vi "Lab Panel V5.12.vi"() -> ()   [LabVIEW 2013] (continued)
                    }
                    n1129 = Increment(x=w2161) -> (x+1=w2162:dbl)
                    n1130 = Greater Or Equal?(x=w2169, y=w2162) -> (x >= y?=w2171:bool)
                    n1131 = case shown="True" w2171 {
                      tunnel: w2166 -> [w2181 _]
                      tunnel: w2165 -> [w2180 _]
                      tunnel: w2164 -> [w2179 _]
                      tunnel: w2163 -> [w2178 _]
                      frame True {
                        n1132 = stacked-sequence {
                          tunnel: w2181 -> [w2185 _]
                          tunnel: w2180 -> [w2183 w2189]
                          tunnel: w2179 -> [_ w2192]
                          tunnel: w2178 -> [w2182 _]
                          frame #0 {
                            n1133 = Build Array(w2183) -> (w2186:string[])
                            n1134 = Build Array(w2185) -> (w2184:dbl[])
                            n1135 = TDMS Write(0:w2182, 5:"TEST PASS", 7:w2186, 9:w2184) -> (15:w2188:errorcluster)  [unwired: 2 in, 3 out]
                            n1136 = local write "data file error"(w2188) -> ()
                          }
                          frame #1 {
                            n1137 = Bundle(cluster=w2192, "STATUS"=w2189) -> (w2190:T4)  [unwired: 2 in]
                            n1138 = local write "RESULT LAB02-1"(TRUE) -> ()
                            n1139 = local write "DISP LAB02-1"(w2190) -> ()
                          }
                        }
                      }
                      frame False {
                      }
                    }
                  }
                }
              }
              frame #3 {
                # "LAB02-2"
                n1140 = Less?(x=w2193, y=2) -> (x < y?=w2196:bool)
                n1141 = local read "DISP LAB02-2"() -> (w2198:T4)
                n1142 = Unbundle(w2198) -> ("STATUS"=w2199:string)  [unwired: 2 out]
                n1143 = Equal?(x=w2199, y="RUN") -> (x = y?=w2195:bool)
                n1144 = And(x=w2195, y=w2196) -> (x .and. y?=w2194:bool)
                n1145 = case shown="True" w2194 {
                  tunnel: w2198 -> [_ w2204]
                  tunnel: w2193 -> [_ w2208]
                  frame False {
                  }
                  frame True {
                    n1146 = local read "SET LAB02-2"() -> (w2210:T5)
                    n1147 = local read "TDMS LAB02-2"() -> (w2203:refnum<k34>)
                    n1148 = Unbundle(w2204) -> ("CYCLE"=w2209:dbl)  [unwired: 2 out]
                    n1149 = Unbundle(w2210) -> ("CYCLES"=w2201:dbl, "T-RISE mins"=w2207:dbl)  [unwired: 3 out]
                    n1150 = case shown="\"T-RISE TEST\"" w2208 {
                      tunnel: w2207 -> [_ _ w2217]
                      tunnel: [w2212 w2214 w2217] -> w2206
                      tunnel: w2201 -> [w2212 w2214 _]
                      tunnel: ["CHART PASS" "CYCLE PASS" "T-RISE PASS"] -> w2205
                      frame "CHART TEST", Default {
                      }
                      frame "CYCLE TEST" {
                      }
                      frame "T-RISE TEST" {
                      }
                    }
                    n1151 = Increment(x=w2201) -> (x+1=w2202:dbl)
                    n1152 = Greater Or Equal?(x=w2209, y=w2202) -> (x >= y?=w2211:bool)
                    n1153 = case shown="True" w2211 {
                      tunnel: w2206 -> [w2221 _]
                      tunnel: w2205 -> [w2220 _]
                      tunnel: w2204 -> [w2219 _]
                      tunnel: w2203 -> [w2218 _]
                      frame True {
                        n1154 = stacked-sequence {
                          tunnel: w2221 -> [w2225 _]
                          tunnel: w2220 -> [w2223 w2229]
                          tunnel: w2219 -> [_ w2232]
                          tunnel: w2218 -> [w2222 _]
                          frame #0 {
                            n1155 = Build Array(w2223) -> (w2226:string[])
                            n1156 = Build Array(w2225) -> (w2224:dbl[])
                            n1157 = TDMS Write(0:w2222, 5:"TEST PASS", 7:w2226, 9:w2224) -> (15:w2228:errorcluster)  [unwired: 2 in, 3 out]
                            n1158 = local write "data file error"(w2228) -> ()
                          }
                          frame #1 {
                            n1159 = Bundle(cluster=w2232, "STATUS"=w2229) -> (w2230:T4)  [unwired: 2 in]
                            n1160 = local write "RESULT LAB02-2"(TRUE) -> ()
                            n1161 = local write "DISP LAB02-2"(w2230) -> ()
                          }
                        }
                      }
                      frame False {
                      }
                    }
                  }
                }
              }
              frame #4 {
                # "LAB03-1"
                n1162 = Less?(x=w2233, y=2) -> (x < y?=w2236:bool)
                n1163 = local read "DISP LAB03-1"() -> (w2238:T4)
                n1164 = Unbundle(w2238) -> ("STATUS"=w2239:string)  [unwired: 2 out]
                n1165 = Equal?(x=w2239, y="RUN") -> (x = y?=w2235:bool)
                n1166 = And(x=w2235, y=w2236) -> (x .and. y?=w2234:bool)
                n1167 = case shown="True" w2234 {
                  tunnel: w2238 -> [_ w2244]
                  tunnel: w2233 -> [_ w2248]
                  frame False {
                  }
                  frame True {
                    n1168 = local read "SET LAB03-1"() -> (w2250:T5)
                    n1169 = local read "TDMS LAB03-1"() -> (w2243:refnum<k34>)
                    n1170 = Unbundle(w2244) -> ("CYCLE"=w2249:dbl)  [unwired: 2 out]
                    n1171 = Unbundle(w2250) -> ("CYCLES"=w2241:dbl, "T-RISE mins"=w2247:dbl)  [unwired: 3 out]
                    n1172 = case shown="\"T-RISE TEST\"" w2248 {
                      tunnel: w2247 -> [_ _ w2257]
                      tunnel: [w2252 w2254 w2257] -> w2246
                      tunnel: w2241 -> [w2252 w2254 _]
                      tunnel: ["CHART PASS" "CYCLE PASS" "T-RISE PASS"] -> w2245
                      frame "CHART TEST", Default {
                      }
                      frame "CYCLE TEST" {
                      }
                      frame "T-RISE TEST" {
                      }
                    }
                    n1173 = Increment(x=w2241) -> (x+1=w2242:dbl)
                    n1174 = Greater Or Equal?(x=w2249, y=w2242) -> (x >= y?=w2251:bool)
                    n1175 = case shown="True" w2251 {
                      tunnel: w2246 -> [w2261 _]
                      tunnel: w2245 -> [w2260 _]
                      tunnel: w2244 -> [w2259 _]
                      tunnel: w2243 -> [w2258 _]
                      frame True {
                        n1176 = stacked-sequence {
                          tunnel: w2261 -> [w2265 _]
                          tunnel: w2260 -> [w2263 w2269]
                          tunnel: w2259 -> [_ w2272]
                          tunnel: w2258 -> [w2262 _]
                          frame #0 {
                            n1177 = Build Array(w2263) -> (w2266:string[])
                            n1178 = Build Array(w2265) -> (w2264:dbl[])
                            n1179 = TDMS Write(0:w2262, 5:"TEST PASS", 7:w2266, 9:w2264) -> (15:w2268:errorcluster)  [unwired: 2 in, 3 out]
                            n1180 = local write "data file error"(w2268) -> ()
                          }
                          frame #1 {
                            n1181 = Bundle(cluster=w2272, "STATUS"=w2269) -> (w2270:T4)  [unwired: 2 in]
                            n1182 = local write "RESULT LAB03-1"(TRUE) -> ()
                            n1183 = local write "DISP LAB03-1"(w2270) -> ()
                          }
                        }
                      }
                      frame False {
                      }
                    }
                  }
                }
              }
              frame #5 {
                # "LAB03-2"
                n1184 = Less?(x=w2273, y=2) -> (x < y?=w2276:bool)
                n1185 = local read "DISP LAB03-2"() -> (w2278:T4)
                n1186 = Unbundle(w2278) -> ("STATUS"=w2279:string)  [unwired: 2 out]
                n1187 = Equal?(x=w2279, y="RUN") -> (x = y?=w2275:bool)
                n1188 = And(x=w2275, y=w2276) -> (x .and. y?=w2274:bool)
                n1189 = case shown="True" w2274 {
                  tunnel: w2278 -> [_ w2284]
                  tunnel: w2273 -> [_ w2288]
                  frame False {
                  }
                  frame True {
                    n1190 = local read "SET LAB03-2"() -> (w2290:T5)
                    n1191 = local read "TDMS LAB03-2"() -> (w2283:refnum<k34>)
                    n1192 = Unbundle(w2284) -> ("CYCLE"=w2289:dbl)  [unwired: 2 out]
                    n1193 = Unbundle(w2290) -> ("CYCLES"=w2281:dbl, "T-RISE mins"=w2287:dbl)  [unwired: 3 out]
                    n1194 = case shown="\"T-RISE TEST\"" w2288 {
                      tunnel: w2287 -> [_ _ w2297]
                      tunnel: [w2292 w2294 w2297] -> w2286
                      tunnel: w2281 -> [w2292 w2294 _]
                      tunnel: ["CHART PASS" "CYCLE PASS" "T-RISE PASS"] -> w2285
                      frame "CHART TEST", Default {
                      }
                      frame "CYCLE TEST" {
                      }
                      frame "T-RISE TEST" {
                      }
                    }
                    n1195 = Increment(x=w2281) -> (x+1=w2282:dbl)
                    n1196 = Greater Or Equal?(x=w2289, y=w2282) -> (x >= y?=w2291:bool)
                    n1197 = case shown="True" w2291 {
                      tunnel: w2286 -> [w2301 _]
                      tunnel: w2285 -> [w2300 _]
                      tunnel: w2284 -> [w2299 _]
                      tunnel: w2283 -> [w2298 _]
                      frame True {
                        n1198 = stacked-sequence {
                          tunnel: w2301 -> [w2305 _]
                          tunnel: w2300 -> [w2303 w2309]
                          tunnel: w2299 -> [_ w2312]
                          tunnel: w2298 -> [w2302 _]
                          frame #0 {
                            n1199 = Build Array(w2303) -> (w2306:string[])
                            n1200 = Build Array(w2305) -> (w2304:dbl[])
                            n1201 = TDMS Write(0:w2302, 5:"TEST PASS", 7:w2306, 9:w2304) -> (15:w2308:errorcluster)  [unwired: 2 in, 3 out]
                            n1202 = local write "data file error"(w2308) -> ()
                          }
                          frame #1 {
                            n1203 = Bundle(cluster=w2312, "STATUS"=w2309) -> (w2310:T4)  [unwired: 2 in]
                            n1204 = local write "RESULT LAB03-2"(TRUE) -> ()
                            n1205 = local write "DISP LAB03-2"(w2310) -> ()
                          }
                        }
                      }
                      frame False {
                      }
                    }
                  }
                }
              }
              frame #6 {
                # "LAB04-1"
                n1206 = Less?(x=w2313, y=2) -> (x < y?=w2316:bool)
                n1207 = local read "DISP LAB04-1"() -> (w2318:T4)
                n1208 = Unbundle(w2318) -> ("STATUS"=w2319:string)  [unwired: 2 out]
                n1209 = Equal?(x=w2319, y="RUN") -> (x = y?=w2315:bool)
                n1210 = And(x=w2315, y=w2316) -> (x .and. y?=w2314:bool)
                n1211 = case shown="True" w2314 {
                  tunnel: w2318 -> [_ w2324]
                  tunnel: w2313 -> [_ w2328]
                  frame False {
                  }
                  frame True {
                    n1212 = local read "SET LAB04-1"() -> (w2330:T5)
                    n1213 = local read "TDMS LAB04-1"() -> (w2323:refnum<k34>)
                    n1214 = Unbundle(w2324) -> ("CYCLE"=w2329:dbl)  [unwired: 2 out]
                    n1215 = Unbundle(w2330) -> ("CYCLES"=w2321:dbl, "T-RISE mins"=w2327:dbl)  [unwired: 3 out]
                    n1216 = case shown="\"T-RISE TEST\"" w2328 {
                      tunnel: w2327 -> [_ _ w2337]
                      tunnel: [w2332 w2334 w2337] -> w2326
                      tunnel: w2321 -> [w2332 w2334 _]
                      tunnel: ["CHART PASS" "CYCLE PASS" "T-RISE PASS"] -> w2325
                      frame "CHART TEST", Default {
                      }
                      frame "CYCLE TEST" {
                      }
                      frame "T-RISE TEST" {
                      }
                    }
                    n1217 = Increment(x=w2321) -> (x+1=w2322:dbl)
                    n1218 = Greater Or Equal?(x=w2329, y=w2322) -> (x >= y?=w2331:bool)
                    n1219 = case shown="True" w2331 {
                      tunnel: w2326 -> [w2341 _]
                      tunnel: w2325 -> [w2340 _]
                      tunnel: w2324 -> [w2339 _]
                      tunnel: w2323 -> [w2338 _]
                      frame True {
                        n1220 = stacked-sequence {
                          tunnel: w2341 -> [w2345 _]
                          tunnel: w2340 -> [w2343 w2349]
                          tunnel: w2339 -> [_ w2352]
                          tunnel: w2338 -> [w2342 _]
                          frame #0 {
                            n1221 = Build Array(w2343) -> (w2346:string[])
                            n1222 = Build Array(w2345) -> (w2344:dbl[])
                            n1223 = TDMS Write(0:w2342, 5:"TEST PASS", 7:w2346, 9:w2344) -> (15:w2348:errorcluster)  [unwired: 2 in, 3 out]
                            n1224 = local write "data file error"(w2348) -> ()
                          }
                          frame #1 {
                            n1225 = Bundle(cluster=w2352, "STATUS"=w2349) -> (w2350:T4)  [unwired: 2 in]
                            n1226 = local write "RESULT LAB04-1"(TRUE) -> ()
                            n1227 = local write "DISP LAB04-1"(w2350) -> ()
                          }
                        }
                      }
                      frame False {
                      }
                    }
                  }
                }
              }
              frame #7 {
                # "LAB04-2"
                n1228 = Less?(x=w2353, y=2) -> (x < y?=w2356:bool)
                n1229 = local read "DISP LAB04-2"() -> (w2358:T4)
                n1230 = Unbundle(w2358) -> ("STATUS"=w2359:string)  [unwired: 2 out]
                n1231 = Equal?(x=w2359, y="RUN") -> (x = y?=w2355:bool)
                n1232 = And(x=w2355, y=w2356) -> (x .and. y?=w2354:bool)
                n1233 = case shown="True" w2354 {
                  tunnel: w2358 -> [_ w2364]
                  tunnel: w2353 -> [_ w2368]
                  frame False {
                  }
                  frame True {
                    n1234 = local read "SET LAB04-2"() -> (w2370:T5)
                    n1235 = local read "TDMS LAB04-2"() -> (w2363:refnum<k34>)
                    n1236 = Unbundle(w2364) -> ("CYCLE"=w2369:dbl)  [unwired: 2 out]
                    n1237 = Unbundle(w2370) -> ("CYCLES"=w2361:dbl, "T-RISE mins"=w2367:dbl)  [unwired: 3 out]
                    n1238 = case shown="\"T-RISE TEST\"" w2368 {
                      tunnel: w2367 -> [_ _ w2377]
                      tunnel: [w2372 w2374 w2377] -> w2366
                      tunnel: w2361 -> [w2372 w2374 _]
                      tunnel: ["CHART PASS" "CYCLE PASS" "T-RISE PASS"] -> w2365
                      frame "CHART TEST", Default {
                      }
                      frame "CYCLE TEST" {
                      }
                      frame "T-RISE TEST" {
                      }
                    }
                    n1239 = Increment(x=w2361) -> (x+1=w2362:dbl)
                    n1240 = Greater Or Equal?(x=w2369, y=w2362) -> (x >= y?=w2371:bool)
                    n1241 = case shown="True" w2371 {
                      tunnel: w2366 -> [w2381 _]
                      tunnel: w2365 -> [w2380 _]
                      tunnel: w2364 -> [w2379 _]
                      tunnel: w2363 -> [w2378 _]
                      frame True {
                        n1242 = stacked-sequence {
                          tunnel: w2381 -> [w2385 _]
                          tunnel: w2380 -> [w2383 w2389]
                          tunnel: w2379 -> [_ w2392]
                          tunnel: w2378 -> [w2382 _]
                          frame #0 {
                            n1243 = Build Array(w2383) -> (w2386:string[])
                            n1244 = Build Array(w2385) -> (w2384:dbl[])
                            n1245 = TDMS Write(0:w2382, 5:"TEST PASS", 7:w2386, 9:w2384) -> (15:w2388:errorcluster)  [unwired: 2 in, 3 out]
                            n1246 = local write "data file error"(w2388) -> ()
                          }
                          frame #1 {
                            n1247 = Bundle(cluster=w2392, "STATUS"=w2389) -> (w2390:T4)  [unwired: 2 in]
                            n1248 = local write "RESULT LAB04-2"(TRUE) -> ()
                            n1249 = local write "DISP LAB04-2"(w2390) -> ()
                          }
                        }
                      }
                      frame False {
                      }
                    }
                  }
                }
              }
              frame #8 {
                # "LAB05-1"
                n1250 = Less?(x=w2393, y=2) -> (x < y?=w2396:bool)
                n1251 = local read "DISP LAB05-1"() -> (w2398:T4)
                n1252 = Unbundle(w2398) -> ("STATUS"=w2399:string)  [unwired: 2 out]
                n1253 = Equal?(x=w2399, y="RUN") -> (x = y?=w2395:bool)
                n1254 = And(x=w2395, y=w2396) -> (x .and. y?=w2394:bool)
                n1255 = case shown="True" w2394 {
                  tunnel: w2398 -> [_ w2404]
                  tunnel: w2393 -> [_ w2408]
                  frame False {
                  }
                  frame True {
                    n1256 = local read "SET LAB05-1"() -> (w2410:T5)
                    n1257 = local read "TDMS LAB05-1"() -> (w2403:refnum<k34>)
                    n1258 = Unbundle(w2404) -> ("CYCLE"=w2409:dbl)  [unwired: 2 out]
                    n1259 = Unbundle(w2410) -> ("CYCLES"=w2401:dbl, "T-RISE mins"=w2407:dbl)  [unwired: 3 out]
                    n1260 = case shown="\"T-RISE TEST\"" w2408 {
                      tunnel: w2407 -> [_ _ w2417]
                      tunnel: [w2412 w2414 w2417] -> w2406
                      tunnel: w2401 -> [w2412 w2414 _]
                      tunnel: ["CHART PASS" "CYCLE PASS" "T-RISE PASS"] -> w2405
                      frame "CHART TEST", Default {
                      }
                      frame "CYCLE TEST" {
                      }
                      frame "T-RISE TEST" {
                      }
                    }
                    n1261 = Increment(x=w2401) -> (x+1=w2402:dbl)
                    n1262 = Greater Or Equal?(x=w2409, y=w2402) -> (x >= y?=w2411:bool)
                    n1263 = case shown="True" w2411 {
                      tunnel: w2406 -> [w2421 _]
                      tunnel: w2405 -> [w2420 _]
                      tunnel: w2404 -> [w2419 _]
                      tunnel: w2403 -> [w2418 _]
                      frame True {
                        n1264 = stacked-sequence {
                          tunnel: w2421 -> [w2425 _]
                          tunnel: w2420 -> [w2423 w2429]
                          tunnel: w2419 -> [_ w2432]
                          tunnel: w2418 -> [w2422 _]
                          frame #0 {
                            n1265 = Build Array(w2423) -> (w2426:string[])
                            n1266 = Build Array(w2425) -> (w2424:dbl[])
                            n1267 = TDMS Write(0:w2422, 5:"TEST PASS", 7:w2426, 9:w2424) -> (15:w2428:errorcluster)  [unwired: 2 in, 3 out]
                            n1268 = local write "data file error"(w2428) -> ()
                          }
                          frame #1 {
                            n1269 = Bundle(cluster=w2432, "STATUS"=w2429) -> (w2430:T4)  [unwired: 2 in]
                            n1270 = local write "RESULT LAB05-1"(TRUE) -> ()
                            n1271 = local write "DISP LAB05-1"(w2430) -> ()
                          }
                        }
                      }
                      frame False {
                      }
                    }
                  }
                }
              }
              frame #9 {
                # "LAB05-2"
                n1272 = Less?(x=w2433, y=2) -> (x < y?=w2436:bool)
                n1273 = local read "DISP LAB05-2"() -> (w2438:T4)
                n1274 = Unbundle(w2438) -> ("STATUS"=w2439:string)  [unwired: 2 out]
                n1275 = Equal?(x=w2439, y="RUN") -> (x = y?=w2435:bool)
                n1276 = And(x=w2435, y=w2436) -> (x .and. y?=w2434:bool)
                n1277 = case shown="True" w2434 {
                  tunnel: w2438 -> [_ w2444]
                  tunnel: w2433 -> [_ w2448]
                  frame False {
                  }
                  frame True {
                    n1278 = local read "SET LAB05-2"() -> (w2450:T5)
                    n1279 = local read "TDMS LAB05-2"() -> (w2443:refnum<k34>)
                    n1280 = Unbundle(w2444) -> ("CYCLE"=w2449:dbl)  [unwired: 2 out]
                    n1281 = Unbundle(w2450) -> ("CYCLES"=w2441:dbl, "T-RISE mins"=w2447:dbl)  [unwired: 3 out]
                    n1282 = case shown="\"T-RISE TEST\"" w2448 {
                      tunnel: w2447 -> [_ _ w2457]
                      tunnel: [w2452 w2454 w2457] -> w2446
                      tunnel: w2441 -> [w2452 w2454 _]
                      tunnel: ["CHART PASS" "CYCLE PASS" "T-RISE PASS"] -> w2445
                      frame "CHART TEST", Default {
                      }
                      frame "CYCLE TEST" {
                      }
                      frame "T-RISE TEST" {
                      }
                    }
                    n1283 = Increment(x=w2441) -> (x+1=w2442:dbl)
                    n1284 = Greater Or Equal?(x=w2449, y=w2442) -> (x >= y?=w2451:bool)
                    n1285 = case shown="True" w2451 {
                      tunnel: w2446 -> [w2461 _]
                      tunnel: w2445 -> [w2460 _]
                      tunnel: w2444 -> [w2459 _]
                      tunnel: w2443 -> [w2458 _]
                      frame True {
                        n1286 = stacked-sequence {
                          tunnel: w2461 -> [w2465 _]
                          tunnel: w2460 -> [w2463 w2469]
                          tunnel: w2459 -> [_ w2472]
                          tunnel: w2458 -> [w2462 _]
                          frame #0 {
                            n1287 = Build Array(w2463) -> (w2466:string[])
                            n1288 = Build Array(w2465) -> (w2464:dbl[])
                            n1289 = TDMS Write(0:w2462, 5:"TEST PASS", 7:w2466, 9:w2464) -> (15:w2468:errorcluster)  [unwired: 2 in, 3 out]
                            n1290 = local write "data file error"(w2468) -> ()
                          }
                          frame #1 {
                            n1291 = Bundle(cluster=w2472, "STATUS"=w2469) -> (w2470:T4)  [unwired: 2 in]
                            n1292 = local write "RESULT LAB05-2"(TRUE) -> ()
                            n1293 = local write "DISP LAB05-2"(w2470) -> ()
                          }
                        }
                      }
                      frame False {
                      }
                    }
                  }
                }
              }
            }
          }
          frame #5 {
            # "check if test cycles reached for temperature rise test"
            n1294 = stacked-sequence {
              tunnel: w2502 -> [_ _ _ _ _ _ _ _ _ _]
              tunnel: w2501 -> [_ _ _ _ _ _ _ _ _ _]
              tunnel: w2500 -> [_ _ _ _ _ _ _ _ _ _]
              tunnel: w2499 -> [_ _ _ _ _ _ _ _ _ _]
              tunnel: w2498 -> [_ _ _ _ _ _ _ _ _ _]
              tunnel: w2497 -> [_ _ _ _ _ _ _ _ _ _]
              tunnel: w2496 -> [_ _ _ _ _ _ _ _ _ _]
              tunnel: w2495 -> [_ _ _ _ _ _ _ _ _ _]
              tunnel: w2494 -> [_ _ _ _ _ _ _ _ _ _]
              tunnel: w2493 -> [_ _ _ _ _ _ _ _ _ _]
              tunnel: w2492 -> [w2508 _ _ _ _ _ _ _ _ _]
              tunnel: w2482 -> [w2503 _ _ _ _ _ _ _ _ _]
              tunnel: w2491 -> [_ w2534 _ _ _ _ _ _ _ _]
              tunnel: w2490 -> [_ _ w2564 _ _ _ _ _ _ _]
              tunnel: w2489 -> [_ _ _ w2594 _ _ _ _ _ _]
              tunnel: w2488 -> [_ _ _ _ w2624 _ _ _ _ _]
              tunnel: w2487 -> [_ _ _ _ _ w2654 _ _ _ _]
              tunnel: w2486 -> [_ _ _ _ _ _ w2684 _ _ _]
              tunnel: w2485 -> [_ _ _ _ _ _ _ w2714 _ _]
              tunnel: w2484 -> [_ _ _ _ _ _ _ _ w2744 _]
              tunnel: w2483 -> [_ _ _ _ _ _ _ _ _ w2774]
              tunnel: w2481 -> [_ w2533 _ _ _ _ _ _ _ _]
              tunnel: w2480 -> [_ _ w2563 _ _ _ _ _ _ _]
              tunnel: w2479 -> [_ _ _ w2593 _ _ _ _ _ _]
              tunnel: w2478 -> [_ _ _ _ w2623 _ _ _ _ _]
              tunnel: w2477 -> [_ _ _ _ _ w2653 _ _ _ _]
              tunnel: w2476 -> [_ _ _ _ _ _ w2683 _ _ _]
              tunnel: w2475 -> [_ _ _ _ _ _ _ w2713 _ _]
              tunnel: w2474 -> [_ _ _ _ _ _ _ _ w2743 _]
              tunnel: w2473 -> [_ _ _ _ _ _ _ _ _ w2773]
              frame #0 {
                # "LAB01-1"
                n1295 = Equal?(x=w2508, y=2) -> (x = y?=w2506:bool)
                n1296 = local read "DISP LAB01-1"() -> (w2509:T4)
                n1297 = Unbundle(w2509) -> ("STATUS"=w2510:string)  [unwired: 2 out]
                n1298 = Equal?(x=w2510, y="RUN") -> (x = y?=w2505:bool)
                n1299 = And(x=w2505, y=w2506) -> (x .and. y?=w2504:bool)
                n1300 = case shown="True" w2504 {
                  tunnel: w2509 -> [_ w2513]
                  tunnel: w2503 -> [_ w2516]
                  frame False {
                  }
                  frame True {
                    n1301 = local read "SET LAB01-1"() -> (w2515:T5)
                    n1302 = local read "TDMS LAB01-1"() -> (w2512:refnum<k34>)
                    n1303 = Unbundle(w2513) -> ("CYCLE"=w2517:dbl)  [unwired: 2 out]
                    n1304 = Unbundle(w2515) -> ("T-RISE mins"=w2514:dbl)  [unwired: 4 out]
                    n1305 = Greater Or Equal?(x=w2517, y=w2516) -> (x >= y?=w2518:bool)
                    n1306 = case shown="True" w2518 {
                      tunnel: w2514 -> [w2521 _]
                      tunnel: w2513 -> [w2520 _]
                      tunnel: w2512 -> [w2519 _]
                      frame True {
                        n1307 = stacked-sequence {
                          tunnel: w2521 -> [w2524 _]
                          tunnel: w2520 -> [_ w2529]
                          tunnel: w2519 -> [w2522 _]
                          frame #0 {
                            n1308 = Build Array("T-RISE") -> (w2526:string[])
                            n1309 = Build Array(w2524) -> (w2525:dbl[])
                            n1310 = TDMS Write(0:w2522, 5:"TEST PASS", 7:w2526, 9:w2525) -> (15:w2528:errorcluster)  [unwired: 2 in, 3 out]
                            n1311 = local write "data file error"(w2528) -> ()
                          }
                          frame #1 {
                            n1312 = Bundle(cluster=w2529, "STATUS"="T-RISE PASS") -> (w2531:T4)  [unwired: 2 in]
                            n1313 = local write "RESULT LAB01-1"(TRUE) -> ()
                            n1314 = local write "DISP LAB01-1"(w2531) -> ()
                          }
                        }
                      }
                      frame False {
                      }
                    }
                  }
                }
              }
              frame #1 {
                # "LAB01-2"
                n1315 = Equal?(x=w2534, y=2) -> (x = y?=w2537:bool)
                n1316 = local read "DISP LAB01-2"() -> (w2539:T4)
                n1317 = Unbundle(w2539) -> ("STATUS"=w2540:string)  [unwired: 2 out]
                n1318 = Equal?(x=w2540, y="RUN") -> (x = y?=w2536:bool)
                n1319 = And(x=w2536, y=w2537) -> (x .and. y?=w2535:bool)
                n1320 = case shown="True" w2535 {
                  tunnel: w2539 -> [_ w2543]
                  tunnel: w2533 -> [_ w2546]
                  frame False {
                  }
                  frame True {
                    n1321 = local read "SET LAB01-2"() -> (w2545:T5)
                    n1322 = local read "TDMS LAB01-2"() -> (w2542:refnum<k34>)
                    n1323 = Unbundle(w2543) -> ("CYCLE"=w2547:dbl)  [unwired: 2 out]
                    n1324 = Unbundle(w2545) -> ("T-RISE mins"=w2544:dbl)  [unwired: 4 out]
                    n1325 = Greater Or Equal?(x=w2547, y=w2546) -> (x >= y?=w2548:bool)
                    n1326 = case shown="True" w2548 {
                      tunnel: w2544 -> [w2551 _]
                      tunnel: w2543 -> [w2550 _]
                      tunnel: w2542 -> [w2549 _]
                      frame True {
                        n1327 = stacked-sequence {
                          tunnel: w2551 -> [w2554 _]
                          tunnel: w2550 -> [_ w2559]
                          tunnel: w2549 -> [w2552 _]
                          frame #0 {
                            n1328 = Build Array("T-RISE") -> (w2556:string[])
                            n1329 = Build Array(w2554) -> (w2555:dbl[])
                            n1330 = TDMS Write(0:w2552, 5:"TEST PASS", 7:w2556, 9:w2555) -> (15:w2558:errorcluster)  [unwired: 2 in, 3 out]
                            n1331 = local write "data file error"(w2558) -> ()
                          }
                          frame #1 {
                            n1332 = Bundle(cluster=w2559, "STATUS"="T-RISE PASS") -> (w2561:T4)  [unwired: 2 in]
                            n1333 = local write "RESULT LAB01-2"(TRUE) -> ()
                            n1334 = local write "DISP LAB01-2"(w2561) -> ()
                          }
                        }
                      }
                      frame False {
                      }
                    }
                  }
                }
              }
              frame #2 {
                # "LAB02-1"
                n1335 = Equal?(x=w2564, y=2) -> (x = y?=w2567:bool)
                n1336 = local read "DISP LAB02-1"() -> (w2569:T4)
                n1337 = Unbundle(w2569) -> ("STATUS"=w2570:string)  [unwired: 2 out]
                n1338 = Equal?(x=w2570, y="RUN") -> (x = y?=w2566:bool)
                n1339 = And(x=w2566, y=w2567) -> (x .and. y?=w2565:bool)
                n1340 = case shown="True" w2565 {
                  tunnel: w2569 -> [_ w2573]
                  tunnel: w2563 -> [_ w2576]
                  frame False {
                  }
                  frame True {
                    n1341 = local read "SET LAB02-1"() -> (w2575:T5)
                    n1342 = local read "TDMS LAB02-1"() -> (w2572:refnum<k34>)
                    n1343 = Unbundle(w2573) -> ("CYCLE"=w2577:dbl)  [unwired: 2 out]
                    n1344 = Unbundle(w2575) -> ("T-RISE mins"=w2574:dbl)  [unwired: 4 out]
                    n1345 = Greater Or Equal?(x=w2577, y=w2576) -> (x >= y?=w2578:bool)
                    n1346 = case shown="True" w2578 {
                      tunnel: w2574 -> [w2581 _]
                      tunnel: w2573 -> [w2580 _]
                      tunnel: w2572 -> [w2579 _]
                      frame True {
                        n1347 = stacked-sequence {
                          tunnel: w2581 -> [w2584 _]
                          tunnel: w2580 -> [_ w2589]
                          tunnel: w2579 -> [w2582 _]
                          frame #0 {
                            n1348 = Build Array("T-RISE") -> (w2586:string[])
                            n1349 = Build Array(w2584) -> (w2585:dbl[])
                            n1350 = TDMS Write(0:w2582, 5:"TEST PASS", 7:w2586, 9:w2585) -> (15:w2588:errorcluster)  [unwired: 2 in, 3 out]
                            n1351 = local write "data file error"(w2588) -> ()
                          }
                          frame #1 {
                            n1352 = Bundle(cluster=w2589, "STATUS"="T-RISE PASS") -> (w2591:T4)  [unwired: 2 in]
                            n1353 = local write "RESULT LAB02-1"(TRUE) -> ()
                            n1354 = local write "DISP LAB02-1"(w2591) -> ()
                          }
                        }
                      }
                      frame False {
                      }
                    }
                  }
                }
              }
              frame #3 {
                # "LAB02-2"
                n1355 = Equal?(x=w2594, y=2) -> (x = y?=w2597:bool)
                n1356 = local read "DISP LAB02-2"() -> (w2599:T4)
                n1357 = Unbundle(w2599) -> ("STATUS"=w2600:string)  [unwired: 2 out]
                n1358 = Equal?(x=w2600, y="RUN") -> (x = y?=w2596:bool)
                n1359 = And(x=w2596, y=w2597) -> (x .and. y?=w2595:bool)
                n1360 = case shown="True" w2595 {
                  tunnel: w2599 -> [_ w2603]
                  tunnel: w2593 -> [_ w2606]
                  frame False {
                  }
                  frame True {
                    n1361 = local read "SET LAB02-2"() -> (w2605:T5)
                    n1362 = local read "TDMS LAB02-2"() -> (w2602:refnum<k34>)
                    n1363 = Unbundle(w2603) -> ("CYCLE"=w2607:dbl)  [unwired: 2 out]
                    n1364 = Unbundle(w2605) -> ("T-RISE mins"=w2604:dbl)  [unwired: 4 out]
                    n1365 = Greater Or Equal?(x=w2607, y=w2606) -> (x >= y?=w2608:bool)
                    n1366 = case shown="True" w2608 {
                      tunnel: w2604 -> [w2611 _]
                      tunnel: w2603 -> [w2610 _]
                      tunnel: w2602 -> [w2609 _]
                      frame True {
                        n1367 = stacked-sequence {
                          tunnel: w2611 -> [w2614 _]
                          tunnel: w2610 -> [_ w2619]
                          tunnel: w2609 -> [w2612 _]
                          frame #0 {
                            n1368 = Build Array("T-RISE") -> (w2616:string[])
                            n1369 = Build Array(w2614) -> (w2615:dbl[])
                            n1370 = TDMS Write(0:w2612, 5:"TEST PASS", 7:w2616, 9:w2615) -> (15:w2618:errorcluster)  [unwired: 2 in, 3 out]
                            n1371 = local write "data file error"(w2618) -> ()
                          }
                          frame #1 {
                            n1372 = Bundle(cluster=w2619, "STATUS"="T-RISE PASS") -> (w2621:T4)  [unwired: 2 in]
                            n1373 = local write "RESULT LAB02-2"(TRUE) -> ()
                            n1374 = local write "DISP LAB02-2"(w2621) -> ()
                          }
                        }
                      }
                      frame False {
                      }
                    }
                  }
                }
              }
              frame #4 {
                # "LAB03-1"
                n1375 = Equal?(x=w2624, y=2) -> (x = y?=w2627:bool)
                n1376 = local read "DISP LAB03-1"() -> (w2629:T4)
                n1377 = Unbundle(w2629) -> ("STATUS"=w2630:string)  [unwired: 2 out]
                n1378 = Equal?(x=w2630, y="RUN") -> (x = y?=w2626:bool)
                n1379 = And(x=w2626, y=w2627) -> (x .and. y?=w2625:bool)
                n1380 = case shown="True" w2625 {
                  tunnel: w2629 -> [_ w2633]
                  tunnel: w2623 -> [_ w2636]
                  frame False {
                  }
                  frame True {
                    n1381 = local read "SET LAB03-1"() -> (w2635:T5)
                    n1382 = local read "TDMS LAB03-1"() -> (w2632:refnum<k34>)
                    n1383 = Unbundle(w2633) -> ("CYCLE"=w2637:dbl)  [unwired: 2 out]
                    n1384 = Unbundle(w2635) -> ("T-RISE mins"=w2634:dbl)  [unwired: 4 out]
                    n1385 = Greater Or Equal?(x=w2637, y=w2636) -> (x >= y?=w2638:bool)
                    n1386 = case shown="True" w2638 {
                      tunnel: w2634 -> [w2641 _]
                      tunnel: w2633 -> [w2640 _]
                      tunnel: w2632 -> [w2639 _]
                      frame True {
                        n1387 = stacked-sequence {
                          tunnel: w2641 -> [w2644 _]
                          tunnel: w2640 -> [_ w2649]
                          tunnel: w2639 -> [w2642 _]
                          frame #0 {
                            n1388 = Build Array("T-RISE") -> (w2646:string[])
                            n1389 = Build Array(w2644) -> (w2645:dbl[])
                            n1390 = TDMS Write(0:w2642, 5:"TEST PASS", 7:w2646, 9:w2645) -> (15:w2648:errorcluster)  [unwired: 2 in, 3 out]
                            n1391 = local write "data file error"(w2648) -> ()
                          }
                          frame #1 {
                            n1392 = Bundle(cluster=w2649, "STATUS"="T-RISE PASS") -> (w2651:T4)  [unwired: 2 in]
                            n1393 = local write "RESULT LAB03-1"(TRUE) -> ()
                            n1394 = local write "DISP LAB03-1"(w2651) -> ()
                          }
                        }
                      }
                      frame False {
                      }
                    }
                  }
                }
              }
              frame #5 {
                # "LAB03-2"
                n1395 = Equal?(x=w2654, y=2) -> (x = y?=w2657:bool)
                n1396 = local read "DISP LAB03-2"() -> (w2659:T4)
                n1397 = Unbundle(w2659) -> ("STATUS"=w2660:string)  [unwired: 2 out]
                n1398 = Equal?(x=w2660, y="RUN") -> (x = y?=w2656:bool)
                n1399 = And(x=w2656, y=w2657) -> (x .and. y?=w2655:bool)
                n1400 = case shown="True" w2655 {
                  tunnel: w2659 -> [_ w2663]
                  tunnel: w2653 -> [_ w2666]
                  frame False {
                  }
                  frame True {
                    n1401 = local read "SET LAB03-2"() -> (w2665:T5)
                    n1402 = local read "TDMS LAB03-2"() -> (w2662:refnum<k34>)
                    n1403 = Unbundle(w2663) -> ("CYCLE"=w2667:dbl)  [unwired: 2 out]
                    n1404 = Unbundle(w2665) -> ("T-RISE mins"=w2664:dbl)  [unwired: 4 out]
                    n1405 = Greater Or Equal?(x=w2667, y=w2666) -> (x >= y?=w2668:bool)
                    n1406 = case shown="True" w2668 {
                      tunnel: w2664 -> [w2671 _]
                      tunnel: w2663 -> [w2670 _]
                      tunnel: w2662 -> [w2669 _]
                      frame True {
                        n1407 = stacked-sequence {
                          tunnel: w2671 -> [w2674 _]
                          tunnel: w2670 -> [_ w2679]
                          tunnel: w2669 -> [w2672 _]
                          frame #0 {
                            n1408 = Build Array("T-RISE") -> (w2676:string[])
                            n1409 = Build Array(w2674) -> (w2675:dbl[])
                            n1410 = TDMS Write(0:w2672, 5:"TEST PASS", 7:w2676, 9:w2675) -> (15:w2678:errorcluster)  [unwired: 2 in, 3 out]
                            n1411 = local write "data file error"(w2678) -> ()
                          }
                          frame #1 {
                            n1412 = Bundle(cluster=w2679, "STATUS"="T-RISE PASS") -> (w2681:T4)  [unwired: 2 in]
                            n1413 = local write "RESULT LAB03-2"(TRUE) -> ()
                            n1414 = local write "DISP LAB03-2"(w2681) -> ()
                          }
                        }
                      }
                      frame False {
                      }
                    }
                  }
                }
              }
              frame #6 {
                # "LAB04-1"
                n1415 = Equal?(x=w2684, y=2) -> (x = y?=w2687:bool)
                n1416 = local read "DISP LAB04-1"() -> (w2689:T4)
                n1417 = Unbundle(w2689) -> ("STATUS"=w2690:string)  [unwired: 2 out]
                n1418 = Equal?(x=w2690, y="RUN") -> (x = y?=w2686:bool)
                n1419 = And(x=w2686, y=w2687) -> (x .and. y?=w2685:bool)
                n1420 = case shown="True" w2685 {
                  tunnel: w2689 -> [_ w2693]
                  tunnel: w2683 -> [_ w2696]
                  frame False {
                  }
                  frame True {
                    n1421 = local read "SET LAB04-1"() -> (w2695:T5)
                    n1422 = local read "TDMS LAB04-1"() -> (w2692:refnum<k34>)
                    n1423 = Unbundle(w2693) -> ("CYCLE"=w2697:dbl)  [unwired: 2 out]
                    n1424 = Unbundle(w2695) -> ("T-RISE mins"=w2694:dbl)  [unwired: 4 out]
                    n1425 = Greater Or Equal?(x=w2697, y=w2696) -> (x >= y?=w2698:bool)
                    n1426 = case shown="True" w2698 {
                      tunnel: w2694 -> [w2701 _]
                      tunnel: w2693 -> [w2700 _]
                      tunnel: w2692 -> [w2699 _]
                      frame True {
                        n1427 = stacked-sequence {
                          tunnel: w2701 -> [w2704 _]
                          tunnel: w2700 -> [_ w2709]
                          tunnel: w2699 -> [w2702 _]
                          frame #0 {
                            n1428 = Build Array("T-RISE") -> (w2706:string[])
                            n1429 = Build Array(w2704) -> (w2705:dbl[])
                            n1430 = TDMS Write(0:w2702, 5:"TEST PASS", 7:w2706, 9:w2705) -> (15:w2708:errorcluster)  [unwired: 2 in, 3 out]
                            n1431 = local write "data file error"(w2708) -> ()
                          }
                          frame #1 {
                            n1432 = Bundle(cluster=w2709, "STATUS"="T-RISE PASS") -> (w2711:T4)  [unwired: 2 in]
                            n1433 = local write "RESULT LAB04-1"(TRUE) -> ()
                            n1434 = local write "DISP LAB04-1"(w2711) -> ()
                          }
                        }
                      }
                      frame False {
                      }
                    }
                  }
                }
              }
              frame #7 {
                # "LAB04-2"
                n1435 = Equal?(x=w2714, y=2) -> (x = y?=w2717:bool)
                n1436 = local read "DISP LAB04-2"() -> (w2719:T4)
                n1437 = Unbundle(w2719) -> ("STATUS"=w2720:string)  [unwired: 2 out]
                n1438 = Equal?(x=w2720, y="RUN") -> (x = y?=w2716:bool)
                n1439 = And(x=w2716, y=w2717) -> (x .and. y?=w2715:bool)
                n1440 = case shown="True" w2715 {
                  tunnel: w2719 -> [_ w2723]
                  tunnel: w2713 -> [_ w2726]
                  frame False {
                  }
                  frame True {
                    n1441 = local read "SET LAB04-2"() -> (w2725:T5)
                    n1442 = local read "TDMS LAB04-2"() -> (w2722:refnum<k34>)
                    n1443 = Unbundle(w2723) -> ("CYCLE"=w2727:dbl)  [unwired: 2 out]
                    n1444 = Unbundle(w2725) -> ("T-RISE mins"=w2724:dbl)  [unwired: 4 out]
                    n1445 = Greater Or Equal?(x=w2727, y=w2726) -> (x >= y?=w2728:bool)
                    n1446 = case shown="True" w2728 {
                      tunnel: w2724 -> [w2731 _]
                      tunnel: w2723 -> [w2730 _]
                      tunnel: w2722 -> [w2729 _]
                      frame True {
                        n1447 = stacked-sequence {
                          tunnel: w2731 -> [w2734 _]
                          tunnel: w2730 -> [_ w2739]
                          tunnel: w2729 -> [w2732 _]
                          frame #0 {
                            n1448 = Build Array("T-RISE") -> (w2736:string[])
                            n1449 = Build Array(w2734) -> (w2735:dbl[])
                            n1450 = TDMS Write(0:w2732, 5:"TEST PASS", 7:w2736, 9:w2735) -> (15:w2738:errorcluster)  [unwired: 2 in, 3 out]
                            n1451 = local write "data file error"(w2738) -> ()
                          }
                          frame #1 {
                            n1452 = Bundle(cluster=w2739, "STATUS"="T-RISE PASS") -> (w2741:T4)  [unwired: 2 in]
                            n1453 = local write "RESULT LAB04-2"(TRUE) -> ()
                            n1454 = local write "DISP LAB04-2"(w2741) -> ()
                          }
                        }
                      }
                      frame False {
                      }
                    }
                  }
                }
              }
              frame #8 {
                # "LAB05-1"
                n1455 = Equal?(x=w2744, y=2) -> (x = y?=w2747:bool)
                n1456 = local read "DISP LAB05-1"() -> (w2749:T4)
                n1457 = Unbundle(w2749) -> ("STATUS"=w2750:string)  [unwired: 2 out]
                n1458 = Equal?(x=w2750, y="RUN") -> (x = y?=w2746:bool)
                n1459 = And(x=w2746, y=w2747) -> (x .and. y?=w2745:bool)
                n1460 = case shown="True" w2745 {
                  tunnel: w2749 -> [_ w2753]
                  tunnel: w2743 -> [_ w2756]
                  frame False {
                  }
                  frame True {
                    n1461 = local read "SET LAB05-1"() -> (w2755:T5)
                    n1462 = local read "TDMS LAB05-1"() -> (w2752:refnum<k34>)
                    n1463 = Unbundle(w2753) -> ("CYCLE"=w2757:dbl)  [unwired: 2 out]
                    n1464 = Unbundle(w2755) -> ("T-RISE mins"=w2754:dbl)  [unwired: 4 out]
                    n1465 = Greater Or Equal?(x=w2757, y=w2756) -> (x >= y?=w2758:bool)
                    n1466 = case shown="True" w2758 {
                      tunnel: w2754 -> [w2761 _]
                      tunnel: w2753 -> [w2760 _]
                      tunnel: w2752 -> [w2759 _]
                      frame True {
                        n1467 = stacked-sequence {
                          tunnel: w2761 -> [w2764 _]
                          tunnel: w2760 -> [_ w2769]
                          tunnel: w2759 -> [w2762 _]
                          frame #0 {
                            n1468 = Build Array("T-RISE") -> (w2766:string[])
                            n1469 = Build Array(w2764) -> (w2765:dbl[])
                            n1470 = TDMS Write(0:w2762, 5:"TEST PASS", 7:w2766, 9:w2765) -> (15:w2768:errorcluster)  [unwired: 2 in, 3 out]
                            n1471 = local write "data file error"(w2768) -> ()
                          }
                          frame #1 {
                            n1472 = Bundle(cluster=w2769, "STATUS"="T-RISE PASS") -> (w2771:T4)  [unwired: 2 in]
                            n1473 = local write "RESULT LAB05-1"(TRUE) -> ()
                            n1474 = local write "DISP LAB05-1"(w2771) -> ()
                          }
                        }
                      }
                      frame False {
                      }
                    }
                  }
                }
              }
              frame #9 {
                # "LAB05-2"
                n1475 = Equal?(x=w2774, y=2) -> (x = y?=w2777:bool)
                n1476 = local read "DISP LAB05-2"() -> (w2779:T4)
                n1477 = Unbundle(w2779) -> ("STATUS"=w2780:string)  [unwired: 2 out]
                n1478 = Equal?(x=w2780, y="RUN") -> (x = y?=w2776:bool)
                n1479 = And(x=w2776, y=w2777) -> (x .and. y?=w2775:bool)
                n1480 = case shown="True" w2775 {
                  tunnel: w2779 -> [_ w2783]
                  tunnel: w2773 -> [_ w2786]
                  frame False {
                  }
                  frame True {
                    n1481 = local read "SET LAB05-2"() -> (w2785:T5)
                    n1482 = local read "TDMS LAB05-2"() -> (w2782:refnum<k34>)
                    n1483 = Unbundle(w2783) -> ("CYCLE"=w2787:dbl)  [unwired: 2 out]
                    n1484 = Unbundle(w2785) -> ("T-RISE mins"=w2784:dbl)  [unwired: 4 out]
                    n1485 = Greater Or Equal?(x=w2787, y=w2786) -> (x >= y?=w2788:bool)
                    n1486 = case shown="True" w2788 {
                      tunnel: w2784 -> [w2791 _]
                      tunnel: w2783 -> [w2790 _]
                      tunnel: w2782 -> [w2789 _]
                      frame True {
                        n1487 = stacked-sequence {
                          tunnel: w2791 -> [w2794 _]
                          tunnel: w2790 -> [_ w2799]
                          tunnel: w2789 -> [w2792 _]
                          frame #0 {
                            n1488 = Build Array("T-RISE") -> (w2796:string[])
                            n1489 = Build Array(w2794) -> (w2795:dbl[])
                            n1490 = TDMS Write(0:w2792, 5:"TEST PASS", 7:w2796, 9:w2795) -> (15:w2798:errorcluster)  [unwired: 2 in, 3 out]
                            n1491 = local write "data file error"(w2798) -> ()
                          }
                          frame #1 {
                            n1492 = Bundle(cluster=w2799, "STATUS"="T-RISE PASS") -> (w2801:T4)  [unwired: 2 in]
                            n1493 = local write "RESULT LAB05-2"(TRUE) -> ()
